vi "Parse Text-Comment-Text.vi"(8 "Error In":errorcluster) -> (0 "Error Out":errorcluster)   [LabVIEW 2018, in "Tests.lvlib" / "Lexer.lvlib"]
uses:
  Lexer.lvlib
  src/Toolkit/Low-Level/Tokens/Text/Text.lvclass
  src/Toolkit/Low-Level/Support/Lex String.vi
  <vilib>/Utility/LVClass/Get LV Class Name.vi
  src/Toolkit/Low-Level/Tokens/Text/API/Read Content.vi
  <vilib>/addons/_JKI Toolkits/Caraya/classes/Assert/Assert Equal_Variant.vi
  <vilib>/addons/_JKI Toolkits/Caraya/classes/Test/Test.lvclass
  <vilib>/addons/_JKI Toolkits/Caraya/classes/Assert/Assert.lvclass
  Tests.lvlib
  src/Toolkit/Low-Level/Tokens/Abstract/Abstract.lvclass
  src/Toolkit/Toolkit.lvlib
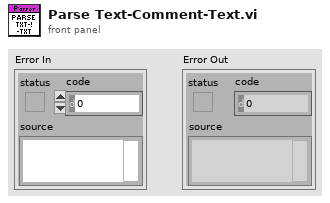
[diagram p1: front panel]
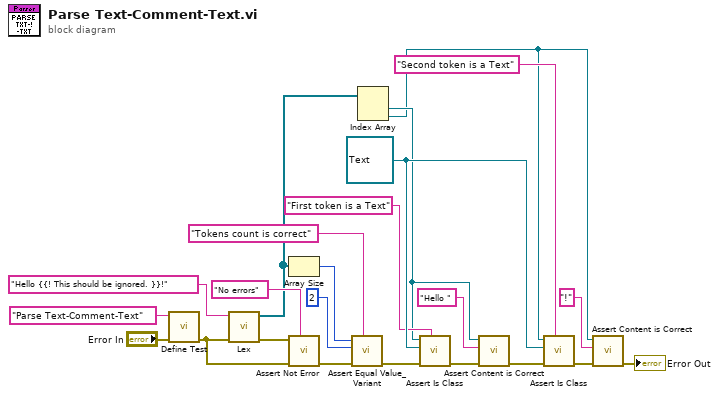
[diagram p0: block diagram]
diagram:
  w9 = refnum<class "Text.lvclass"> refnum ("Mustache.lvlib:Tokens.lvlib:Text.lvclass")
  n1 = call <vilib>:"Define Test.vi"("error in (no error)"="Error In", "Label (VI Title)"="Parse Text-Comment-Text") -> ("error out"=w1:errorcluster)  [unwired: 9 in]
  n2 = call-poly "Lex.vi"("Error In"=w1, "Input"="Hello {{! This should be ignored. }}!" ("format string")) -> ("Error Out"=w21:errorcluster, "Tokens"=w14:refnum<class "Abstract.lvclass">[])  [unwired: 8 in]
  n3 = Array Size(array=w14) -> (size(s)=w17:i32)
  n4 = call <vilib>:"Assert Not Error.vi"("Label"="No errors", "error in (no error)"=w1, "Not Error?"=w21) -> ("error out"=w19:errorcluster)  [unwired: 8 in]
  n5 = call <vilib>:"Assert Equal Value_Variant.vi"("Label"="Tokens count is correct", "error in (no error)"=w19, "Y"=2 ("size(s)"), "X"=w17) -> ("error out"=w15:errorcluster)  [unwired: 7 in]
  n6 = Index Array(array=w14) -> (element #1=w4:refnum<class "Abstract.lvclass">, element #2=w3:refnum<class "Abstract.lvclass">)  [unwired: 2 in]
  n7 = call "Assert Is Class.vi"("Label"="First token is a Text", "Error In"=w15, "Expected"=w9, "Actual"=w4) -> ("Error Out"=w13:errorcluster)  [unwired: 7 in]
  n8 = call "Assert Content is Correct.vi"("Error In"=w13, "Expected"="Hello ", "Token"=w4) -> ("Error Out"=w12:errorcluster)  [unwired: 8 in]
  n9 = call "Assert Is Class.vi"("Label"="Second token is a Text", "Error In"=w12, "Expected"=w9, "Actual"=w3) -> ("Error Out"=w11:errorcluster)  [unwired: 7 in]
  n10 = call "Assert Content is Correct.vi"("Error In"=w11, "Expected"="!", "Token"=w3) -> ("Error Out"=→"Error Out":errorcluster)  [unwired: 8 in]
